vi "Init.vi"(8 "error in (no error)":errorcluster, 11 "Data in":refnum<class "Boolean_1D.lvclass">) -> (0 "error out":errorcluster, 3 "Data out":refnum<class "Boolean_1D.lvclass">)   [LabVIEW 2021, in "Boolean_1D.lvclass"]
uses:
  Boolean_1D.lvclass
  Boolean_1D.lvclass/Boolean_1D.ctl
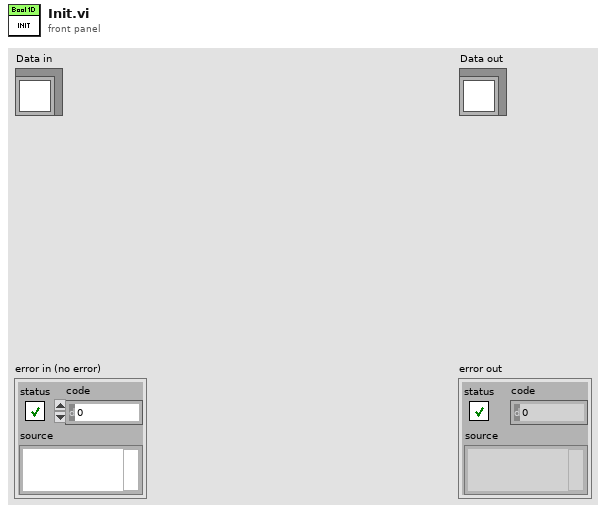
[diagram p1: front panel]
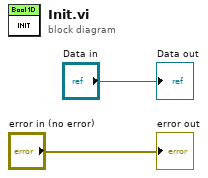
[diagram p0: block diagram]
diagram:
  "error out" <- "error in (no error)"
  "Data out" <- "Data in"
